vi "Beta Inverse CDF.vi"(9 "b":dbl=4.0, 10 "a":dbl=2.0, 11 "cdf(x)":dbl=0.8125) -> (0 "error":i32, 3 "x":dbl=0.500000005)   [LabVIEW 2020, in "NI_Gmath.lvlib"]
doc: "Computes the continuous inverse cumulative distribution function (CDF) of the various distributions. You must manually select the polymorphic instance to use."
uses:
  <vilib>/gmath/NI_Gmath.lvlib
  <vilib>/gmath/statdist.llb/st_error_code.ctl
panel:
  # "Beta Inverse CDF"
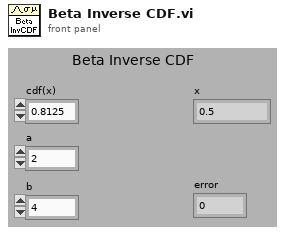
[diagram p1: front panel]
types:
  T1 = typedef "NI_Gmath.lvlib/st_error_code.ctl" = i32
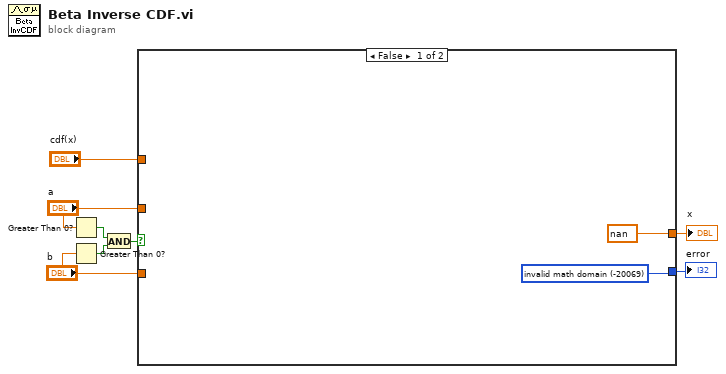
[diagram p0: block diagram]
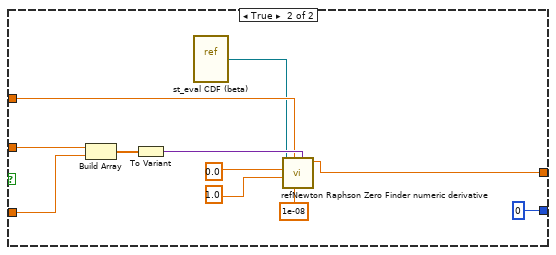
[diagram p2: hidden frame]
diagram:
  n1 = Greater Than 0?(x="a") -> (x > 0?=w4:bool)
  n2 = Greater Than 0?(x="b") -> (x > 0?=w5:bool)
  n3 = And(x=w4, y=w5) -> (x .and. y?=w1:bool)
  n4 = case shown="False" w1 {
    tunnel: "b" -> [_ w17]
    tunnel: [w9 0 ("invalid math domain")] -> w8
    tunnel: [nan w16] -> w7
    tunnel: "cdf(x)" -> [_ w15]
    tunnel: "a" -> [_ w18]
    frame False {
      w9 = T1 -20069 items=["invalid math domain"=-20069, "Fourier interpolation size m >= n"=-20070, "empty array"=-20003] ("stat interp error code")
    }
    frame True {
      n5 = Build Array(w18, w17) -> (w20:dbl[])
      n6 = To Variant(anything=w20) -> (Variant=w19:variant)
      n7 = vi-ref <vilib>:"st_eval CDF (beta).vi"() -> ("vi reference"=w14:refnum<vi>)
      n8 = call <vilib>:"refNewton Raphson Zero Finder numeric derivative.vi"("function parameters"=w19, "accuracy"=1e-08, "level"=w15, "end"=1.0 ("upper limit"), "start"=0.0 ("upper limit"), "function refnum"=w14) -> ("zero"=w16:dbl)  [unwired: 2 in, 3 out]
    }
  }
  "x" <- w7
  "error" <- w8
